vi "Get_Registers.vi"(3 "error in (no error)":errorcluster, 5 "VISA in":refnum<visa-resource-name>) -> (0 "error out":errorcluster, 1 "Registers":T1 {"Reg1" format="0x%08x"; "Reg2" format="0x%08x"; "Reg3" format="0x%08x"; "Reg4" format="0x%08x"; "Reg5" format="0x%08x"; "Reg0" format="0x%08x"; "Reg6" format="0x%08x"}, 2 "VISA out":refnum<visa-resource-name>)   [LabVIEW 2017, in "GP22_TDC_Arduinoed.lvlib"]
doc: "Gets the GP22's internal registers to the given values."
uses:
  GP22_TDC_Arduinoed.lvlib
  Globals.vi
  Registers.ctl
panel:
  out "read buffer":string
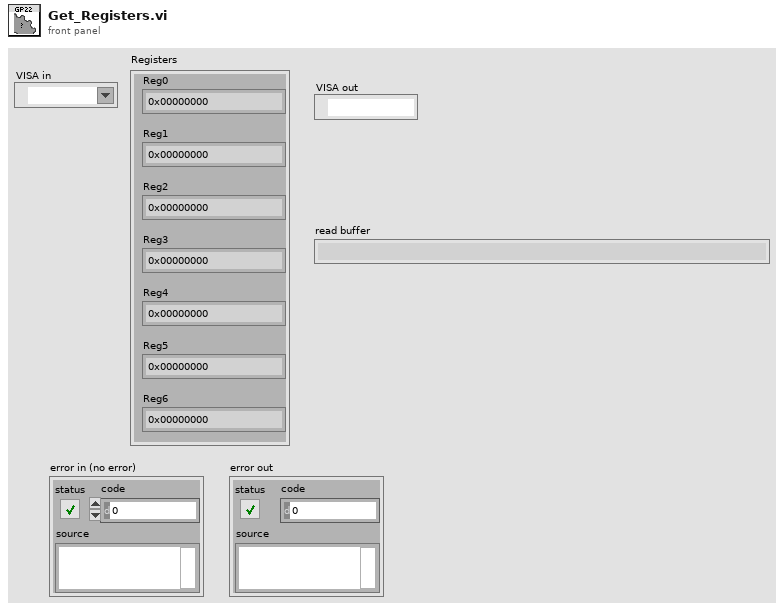
[diagram p1: front panel]
types:
  T1 = typedef "Registers.ctl" = cluster{"Reg0":u32, "Reg1":u32, "Reg2":u32, "Reg3":u32, "Reg4":u32, "Reg5":u32, "Reg6":u32}
  T2 = cluster{"[0]":u32, "[1]":u32, "[2]":u32, "[3]":u32, "[4]":u32, "[5]":u32, "[6]":u32}
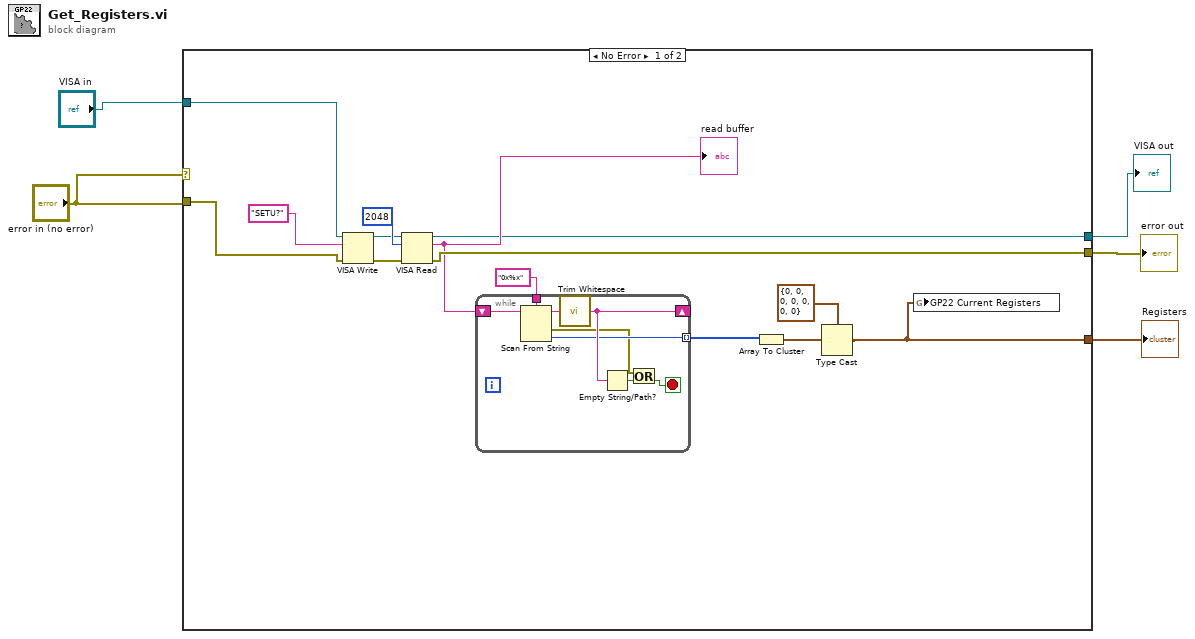
[diagram p0: block diagram]
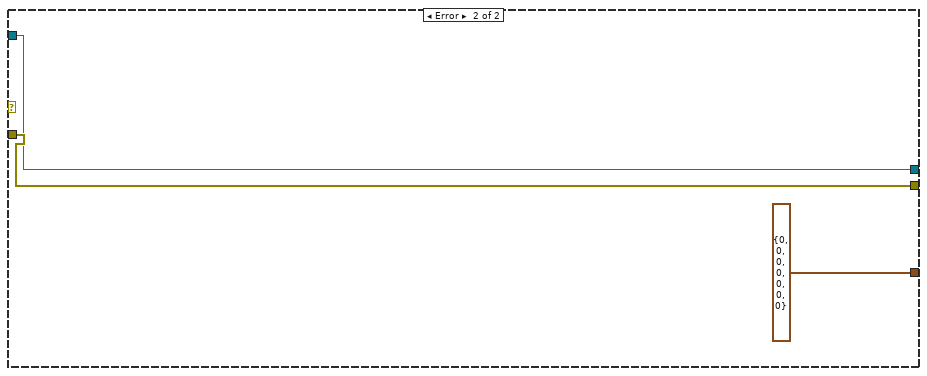
[diagram p2: hidden frame]
diagram:
  n1 = case shown="No Error" "error in (no error)" {
    tunnel: [w15 w30] -> w5
    tunnel: "error in (no error)" -> [w12 w30]
    tunnel: "VISA in" -> [w11 w29]
    tunnel: [w10 w29] -> w2
    tunnel: [w6 T2 {"[0]"=0, "[1]"=0, "[2]"=0, "[3]"=0, "[4]"=0, "[5]"=0, "[6]"=0}] -> w1
    frame No Error {
      n2 = VISA Write(VISA resource name=w11, write buffer="SETU?" ("initial string"), error in (no error)=w12) -> (VISA resource name out=w17:refnum<visa-resource-name>, error out=w18:errorcluster)  [unwired: 1 out]
      n3 = VISA Read(VISA resource name=w17, byte count=u32 2048, error in (no error)=w18) -> (VISA resource name out=w10:refnum<visa-resource-name>, read buffer=w13:string, error out=w15:errorcluster)  [unwired: 1 out]
      "read buffer" <- w13
      n4 = while {
        tunnel: "0x%x" ("format string") -> [w27]
        shift-right: [w23] -> _
        shift-left: w13 -> [w26]
        tunnel: [w22] -> w9 mode=indexing
        stop <- w21 stop-if-true
        n5 = Scan From String(format string=w27, input string=w26) -> (remaining string=w25:string, error out=w20:errorcluster, output 1=w22:u32)  [unwired: 3 in, 1 out]
        n6 = call <vilib>:"Trim Whitespace.vi"("string"=w25) -> ("trimmed string"=w23:string)  [unwired: 1 in]
        n7 = Empty String/Path?(string/path=w23) -> (empty?=w24:bool)
        n8 = Or(x=w20, y=w24) -> (x .or. y?=w21:bool)
      }
      n9 = Array To Cluster(array=w9) -> (cluster=w8:T2)
      n10 = Type Cast(type=T1 {"Reg0"=0, "Reg1"=0, "Reg2"=0, "Reg3"=0, "Reg4"=0, "Reg5"=0, "Reg6"=0} ("Registers"), x=w8) -> (*(type *) &x=w6:T1)
      n11 = global write "Globals.vi" "GP22 Current Registers"(w6) -> ()
    }
    frame Error {
    }
  }
  "error out" <- w5
  "VISA out" <- w2
  "Registers" <- w1
